vi "FRCts20_Backend_ExecSql.vi"(8 "error in (no error)":errorcluster, 10 "format string":string, 11 "Refnum in":T1) -> (0 "error out":errorcluster, 2 "rows affected":i32, 3 "recordset data":variant[][](array[variant]))   [LabVIEW 2013, in "FRCts20_Backend_Engine.lvlib"]
doc: "Excutes a single SQL command and returns the recordset, if needed."
uses:
  FRCts20_Backend_Engine.lvlib
  <vilib>/addons/database/Connection.llb/Conn ObjectReference.ctl
  <vilib>/addons/database/Recordset.llb/Rec Destroy - Connection.vi
  <vilib>/addons/database/Recordset.llb/Rec Fetch Recordset Data (R).vi
  <vilib>/addons/database/NI_Database_API.lvlib
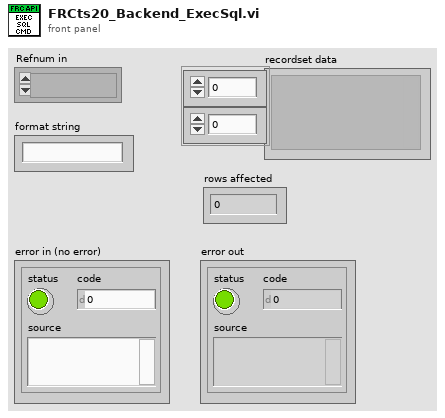
[diagram p1: front panel]
types:
  T1 = typedef "NI_Database_API.lvlib/Conn ObjectReference.ctl" = refnum<k1>
  T2 = typedef "NI_Database_API.lvlib/Rec ObjectReference.ctl" = refnum<k1>
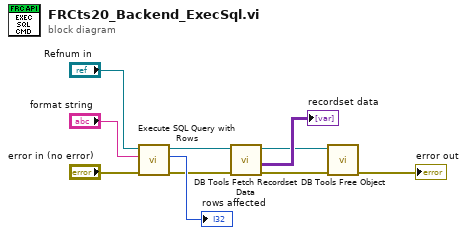
[diagram p0: block diagram]
diagram:
  n1 = call "Execute SQL Query with Rows.vi"("error in (no error)"="error in (no error)", "SQL query"="format string", "connection reference"="Refnum in") -> ("error out"=w6:errorcluster, "rows affected"=→"rows affected":i32, "recordset reference"=w5:T2)  [unwired: 4 in]
  n2 = call-poly <vilib>:"DB Tools Fetch Recordset Data.vi"("error in (no error)"=w6, "recordset reference"=w5) -> ("error out"=w2:errorcluster, "recordset data"=→"recordset data":variant[][], "recordset reference out"=w1:T2)  [unwired: 3 in]
  n3 = call-poly <vilib>:"DB Tools Free Object.vi"("error in (no error)"=w2, "recordset reference"=w1) -> ("error out"=→"error out":errorcluster)  [unwired: 8 in, 1 out]
